vi "GetMethodDependency.vi"(0 "ClassReader in":refnum<class "ClassReader.lvclass">, 1 "Method(s)":variant, 5 "error in (no error)":errorcluster) -> (14 "ClassReader out":refnum<class "ClassReader.lvclass">, 15 "DependencyVIs":T1[](array[typedef]), 19 "error out":errorcluster)   [LabVIEW 2020, in "ClassReader.lvclass"]
uses:
  <resource>/Framework/Providers/Open_GDS/ClassProviders/Provider_BaseClassInterface/ClassReader_class/ClassReader.lvclass
  <resource>/Framework/Providers/Open_GDS/ClassProviders/Provider_BaseClassInterface/ClassReader_class/MethodDependencyType.ctl
  <resource>/Framework/Providers/Open_GDS/ClassProviders/Common/ScriptingFunctions/SubVIs/Scripting_ViDependencyType.ctl
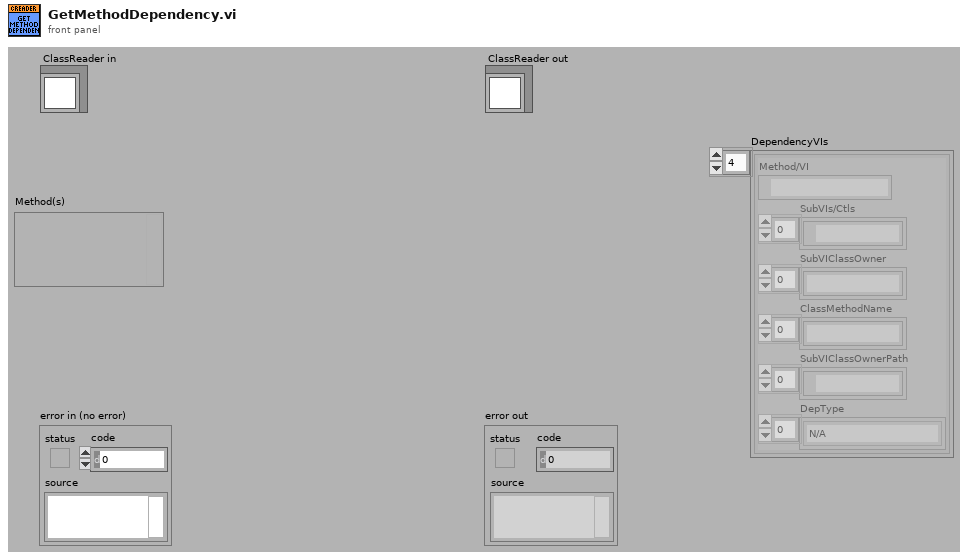
[diagram p1: front panel]
types:
  T1 = typedef "MethodDependencyType.ctl" = cluster{"Method/VI":path, "SubVIs/Ctls":path[], "SubVIClassOwner":string[], "ClassMethodName":string[], "SubVIClassOwnerPath":path[], "DepType":T2[]}
  T2 = typedef "Scripting_ViDependencyType.ctl" = enum16{"N/A", "Launches"}
  T3 = typedef "Scripting_VIClassDependency.ctl" = cluster{"VIPath":path, "Class":string, "ClassPath":path, "ViDependencyType":T2}
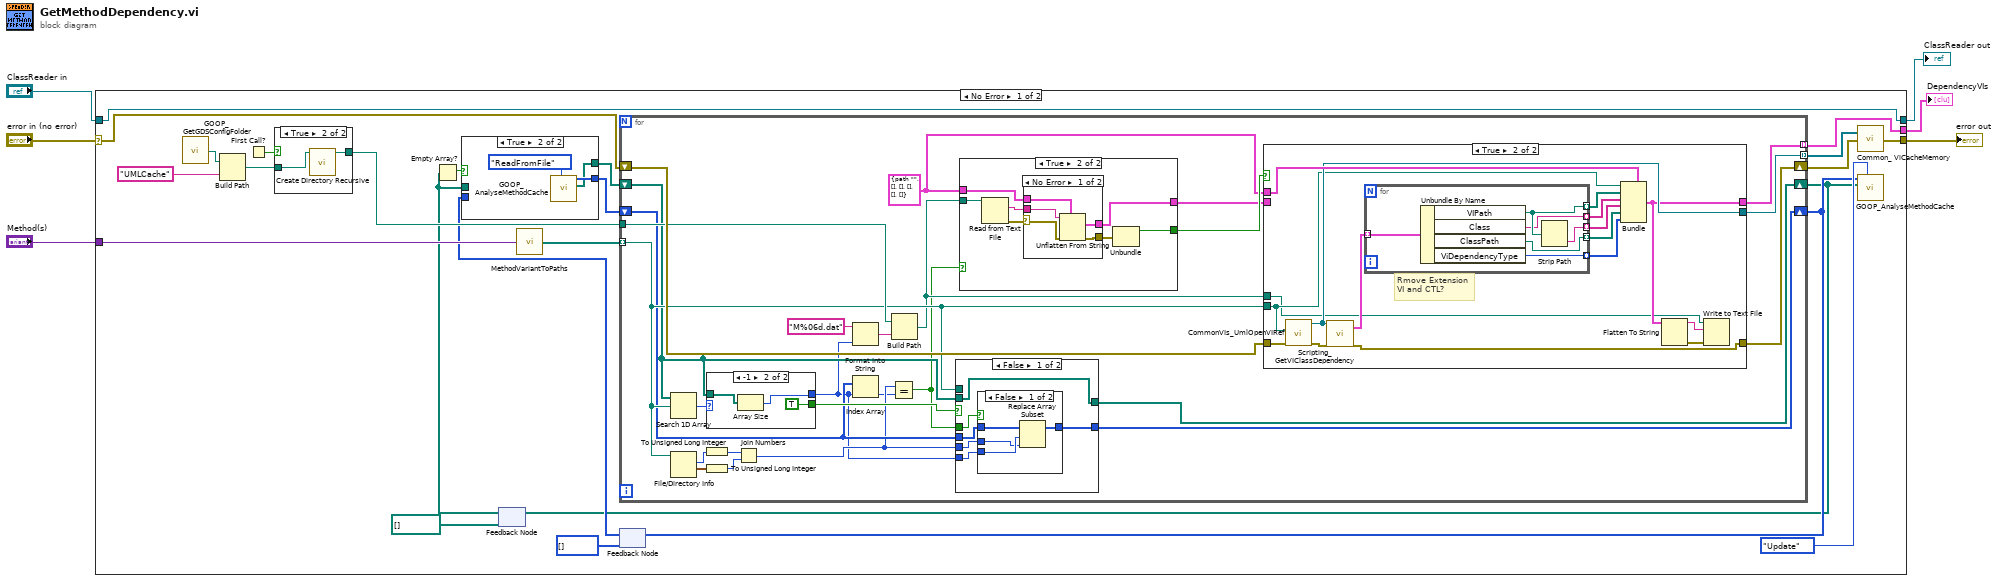
[diagram p0: block diagram]
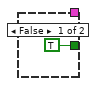
[diagram p4: hidden frame]
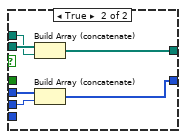
[diagram p7: hidden frame]
diagram:
  n1 = case shown="No Error" "error in (no error)" {
    selector: "error in (no error)" -> [w24 w124]
    tunnel: [w27 w124] -> w5
    tunnel: [w23 w123] -> w3
    tunnel: "ClassReader in" -> [w23 w123]
    tunnel: "Method(s)" -> [w25 _]
    tunnel: [w22 _] -> w1
    frame No Error {
      n2 = call <resource>:"GOOP_GetGDSConfigFolder.vi"() -> ("GDSFolderPath"=w21:path)
      n3 = Build Path(base path=w21, name or relative path="UMLCache") -> (appended path=w18:path)
      n4 = First Call?() -> (First Call?: T/F=w19:bool)
      n5 = case shown="True" w19 {
        tunnel: w18 -> [w35 w37]
        tunnel: [w35 w36] -> w17
        frame False {
        }
        frame True {
          n6 = call <vilib>:"Create Directory Recursive.vi"("directory"=w37) -> ("directory copy"=w36:path)  [unwired: 4 in, 2 out]
        }
      }
      n7 = feedback #1(path[] [] ("Paths")) -> (w13:path[])
      n8 = Empty Array?(array=w13) -> (empty?=w14:bool)
      n9 = call <resource>:"MethodVariantToPaths.vi"("Method(s)"=w25) -> ("Paths"=w26:path[])
      n10 = feedback #2(u64[] [] ("Paths")) -> (w11:u64[])
      n11 = case shown="True" w14 {
        tunnel: w13 -> [w31 _]
        tunnel: [w31 w33] -> w12
        tunnel: w11 -> [w30 _]
        tunnel: [w30 w34] -> w10
        frame False {
        }
        frame True {
          n12 = call <resource>:"GOOP_AnalyseMethodCache.vi"("Actions"=enum16{"Update", "ReadFromFile", "SaveToFile"}."ReadFromFile") -> ("PathsOut"=w33:path[], "Date And Size ID(U64)Out"=w34:u64[])  [unwired: 8 in, 1 out]
        }
      }
      n13 = for {
        shift-right: [w62] -> w29
        shift-left: w24 -> [w63]
        tunnel: [w61] -> w28 mode=indexing
        tunnel: w26 -> [w46] mode=indexing
        tunnel: [w60] -> w22 mode=indexing
        tunnel: w17 -> [w59]
        shift-right: [w54] -> w7
        shift-left: w12 -> [w41]
        shift-right: [w49] -> w8
        shift-left: w10 -> [w45]
        w38 = T1 {"Method/VI"=path "", "SubVIs/Ctls"=[], "SubVIClassOwner"=[], "ClassMethodName"=[], "SubVIClassOwnerPath"=[], "DepType"=[]}
        n14 = Search 1D Array(1D array=w41, element=w46) -> (index of element=w56:i32)  [unwired: 1 in]
        n15 = File/Directory Info(path=w46) -> (size=w52:i64, last mod=w53:timestamp)  [unwired: 1 in, 5 out]
        n16 = To Unsigned Long Integer(number=w52) -> (unsigned 32bit integer=w51:u32)
        n17 = To Unsigned Long Integer(number=w53) -> (unsigned 32bit integer=w50:u32)
        n18 = case shown="-1" w56 {
          selector: w56 -> [w95 _]
          tunnel: [_ TRUE] -> w55
          tunnel: [w95 w96] -> w39
          tunnel: w41 -> [_ w97]
          frame 0, Default {
          }
          frame -1 {
            n19 = Array Size(array=w97) -> (size(s)=w96:i32)
          }
        }
        n20 = Join Numbers(hi=w51, lo=w50) -> ((hi.lo)=w44:u64)
        n21 = Format Into String(format string="M%06d.dat", w39) -> (resulting string=w47:string)  [unwired: 2 in, 1 out]
        n22 = Index Array(array=w45, index=w39) -> (element=w43:u64)
        n23 = Equal?(x=w44, y=w43) -> (x = y?=w40:bool)
        n24 = Build Path(base path=w59, name or relative path=w47) -> (appended path=w42:path)
        n25 = case shown="False" w55 {
          tunnel: w41 -> [w83 w94]
          tunnel: [w83 w93] -> w54
          tunnel: w46 -> [_ w92]
          tunnel: w45 -> [w81 w89]
          tunnel: [w80 w90] -> w49
          tunnel: w44 -> [w78 w91]
          tunnel: w40 -> [w82 _]
          tunnel: w39 -> [w79 _]
          frame False {
            n26 = case shown="False" w82 {
              tunnel: w81 -> [w87 w88]
              tunnel: [w86 w88] -> w80
              tunnel: w79 -> [w85 _]
              tunnel: w78 -> [w84 _]
              frame False {
                n27 = Replace Array Subset(array=w87, new element=w84, index=w85) -> (w86:u64[])
              }
              frame True {
              }
            }
          }
          frame True {
            n28 = Build Array (concatenate)(w94, w92) -> (w93:path[])
            n29 = Build Array (concatenate)(w89, w91) -> (w90:u64[])
          }
        }
        n30 = case shown="True" w40 {
          tunnel: [TRUE ("status") w65] -> w58
          tunnel: w38 -> [_ w69]
          tunnel: [_ w68] -> w57
          tunnel: w42 -> [_ w67]
          frame False {
          }
          frame True {
            n31 = Read from Text File(file (use dialog)=w67) -> (text=w70:string, error out=w71:errorcluster)  [unwired: 3 in, 2 out]
            n32 = case shown="No Error" w71 {
              selector: w71 -> [w76 w77]
              tunnel: [w75 w77] -> w66
              tunnel: w70 -> [w74 _]
              tunnel: w69 -> [w73 _]
              tunnel: [w72 _] -> w68
              frame No Error {
                n33 = Unflatten From String(type=w73, binary string=w74, error in (no error)=w76) -> (value=w72:T1, error out=w75:errorcluster)  [unwired: 2 in, 1 out]
              }
              frame Error {
              }
            }
            n34 = Unbundle(w66) -> ("status"=w65:bool)  [unwired: 2 out]
          }
        }
        n35 = case shown="True" w58 {
          tunnel: w38 -> [_ w116]
          tunnel: w63 -> [w99 w114]
          tunnel: [w99 w108] -> w62
          tunnel: [_ w107] -> w61
          tunnel: [w100 w104] -> w60
          tunnel: w46 -> [_ w105]
          tunnel: w57 -> [w100 _]
          tunnel: w42 -> [_ w102]
          frame False {
          }
          frame True {
            # "Rmove Extension\nVI and CTL?"
            n36 = call <resource>:"CommonVIs_UmlOpenVIRef.vi"("error in"=w114, "ViPath/ViName"=w105) -> ("error out"=w113:errorcluster, "vi reference"=w107:refnum<vi>)  [unwired: 6 in, 2 out]
            n37 = call <resource>:"Scripting_GetVIClassDependency.vi"("ViRef"=w107, "error in (no error)"=w113) -> ("DepVIs"=w115:T3[], "error out"=w108:errorcluster)  [unwired: 16 in]
            n38 = for {
              tunnel: w115 -> [w122] mode=indexing
              tunnel: [w121] -> w112 mode=indexing
              tunnel: [w120] -> w111 mode=indexing
              tunnel: [w119] -> w110 mode=indexing
              tunnel: [w118] -> w109 mode=indexing
              tunnel: [w117] -> w106 mode=indexing
              n39 = Unbundle By Name(w122) -> ("VIPath"=w121:path, "Class"=w120:string, "ClassPath"=w118:path, "ViDependencyType"=w117:T2)
              n40 = Strip Path(path=w121) -> (name=w119:string)  [unwired: 1 out]
            }
            n41 = Bundle(cluster=w116, "Method/VI"=w105, "SubVIs/Ctls"=w112, "SubVIClassOwner"=w111, "ClassMethodName"=w110, "SubVIClassOwnerPath"=w109, "DepType"=w106) -> (w104:T1)
            n42 = Flatten To String(anything=w104) -> (data string=w101:string, error out=w103:errorcluster)  [unwired: 3 in, 1 out]
            n43 = Write to Text File(file (use dialog)=w102, text=w101, error in=w103) -> ()  [unwired: 1 in, 3 out]
          }
        }
      }
      n44 = feedback-in #1(w7) -> ()
      n45 = feedback-in #2(w8) -> ()
      n46 = call <resource>:"Common_ ViCacheMemory.vi"("ViRef-Array"=w28, "error in (no error)"=w29) -> ("error out"=w27:errorcluster)  [unwired: 17 in]
      n47 = call <resource>:"GOOP_AnalyseMethodCache.vi"("Actions"=enum16{"Update", "ReadFromFile", "SaveToFile"}."Update", "Paths"=w7, "Date And Size ID(U64)"=w8) -> ()  [unwired: 6 in, 3 out]
    }
    frame Error {
    }
  }
  "error out" <- w5
  "ClassReader out" <- w3
  "DependencyVIs" <- w1
